vi "Variant to String.vi"(8 "error in (no error)":errorcluster, 10 "Variant":variant, 11 "Numeric Value in":refnum<class "Numeric Value.lvclass">) -> (0 "error out":errorcluster, 2 "String":string, 3 "Numeric Value out":refnum<class "Numeric Value.lvclass">)   [LabVIEW 2020, in "Composed Columns.lvlib" / "Numeric Value.lvclass"]
uses:
  Numeric Value.lvclass
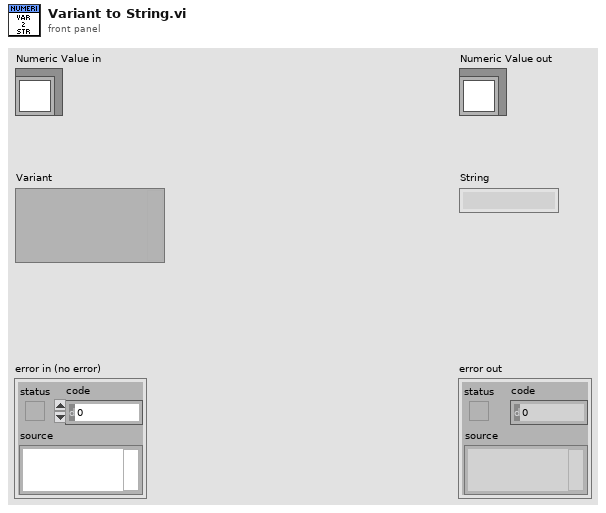
[diagram p1: front panel]
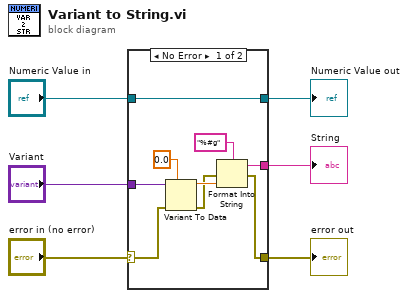
[diagram p0: block diagram]
diagram:
  n1 = case shown="No Error" "error in (no error)" {
    selector: "error in (no error)" -> [w13 w17]
    tunnel: "Numeric Value in" -> [w12 w16]
    tunnel: [w7 w17] -> w4
    tunnel: [w12 w16] -> w3
    tunnel: "Variant" -> [w15 _]
    tunnel: [w9 _] -> w1
    frame No Error {
      n2 = Variant To Data(error in=w13, type=0.0, Variant=w15) -> (data=w10:dbl, error out=w8:errorcluster)
      n3 = Format Into String(format string="%#g", error in=w8, w10) -> (resulting string=w9:string, error out=w7:errorcluster)  [unwired: 1 in]
    }
    frame Error {
    }
  }
  "error out" <- w4
  "Numeric Value out" <- w3
  "String" <- w1
